vi "SRV_Is Not Equal to Zero.vi"(7 "Numeric (DBL)":dbl) -> (8 "Not Zero":bool)   [LabVIEW 2009]
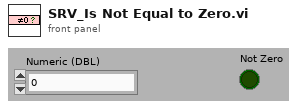
[diagram p1: front panel]
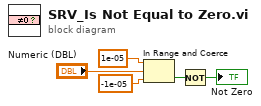
[diagram p0: block diagram]
diagram:
  n1 = In Range and Coerce(upper limit=1e-05, x="Numeric (DBL)", lower limit=-1e-05 ("upper limit")) -> (In Range?=w5:bool)  [unwired: 1 out]
  n2 = Not(x=w5) -> (.not. x?=→"Not Zero":bool)
